vi "excelBinDataMT1.vi"(5 "step":string, 6 "start row":i32, 7 "jobno":string, 8 "error in (no error) 2":errorcluster, 9 "report in":refnum<class "NI_report.lvclass">, 10 "error in (no error)":errorcluster, 11 "connection reference 2":T1) -> (0 "error out 2":errorcluster, 1 "report out":refnum<class "NI_report.lvclass">, 2 "error out":errorcluster, 3 "connection reference":T1)   [LabVIEW 2012]
uses:
  <vilib>/addons/database/Connection.llb/Conn ObjectReference.ctl
  <vilib>/Utility/NIReport.llb/NI_report.lvclass
  <vilib>/addons/database/Auxilliary.llb/DB Tools Cursor Type.ctl
  <vilib>/addons/database/Connection.llb/Conn Execute.vi
  <vilib>/addons/database/Recordset.llb/Rec Fetch String Data (R).vi
  <vilib>/addons/database/Recordset.llb/Rec Fetch Integer Data (R).vi
  <vilib>/addons/database/Recordset.llb/Rec Destroy - Connection.vi
  <vilib>/addons/database/NI_Database_API.lvlib
  <vilib>/Utility/NIReport.llb/Excel/NI_Excel.lvclass
panel:
  in  "start (0, 0)":cluster{"start row":i32, "start column":i32}
  out "concatenated string":string
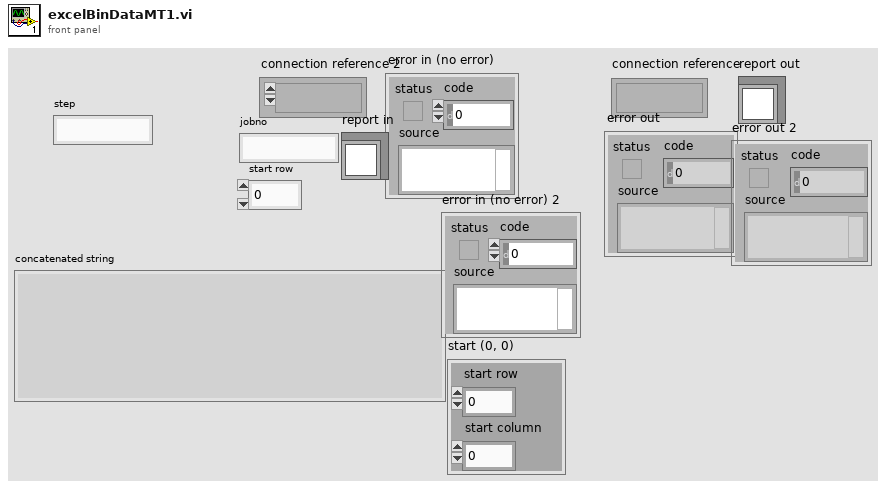
[diagram p1: front panel]
types:
  T1 = typedef "NI_Database_API.lvlib/Conn ObjectReference.ctl" = refnum<k1>
  T2 = typedef "NI_Database_API.lvlib/DB Tools Cursor Type.ctl" = enum16{"forward-only", "keyset", "dynamic", "static"}
  T3 = typedef "NI_Database_API.lvlib/Rec ObjectReference.ctl" = refnum<k1>
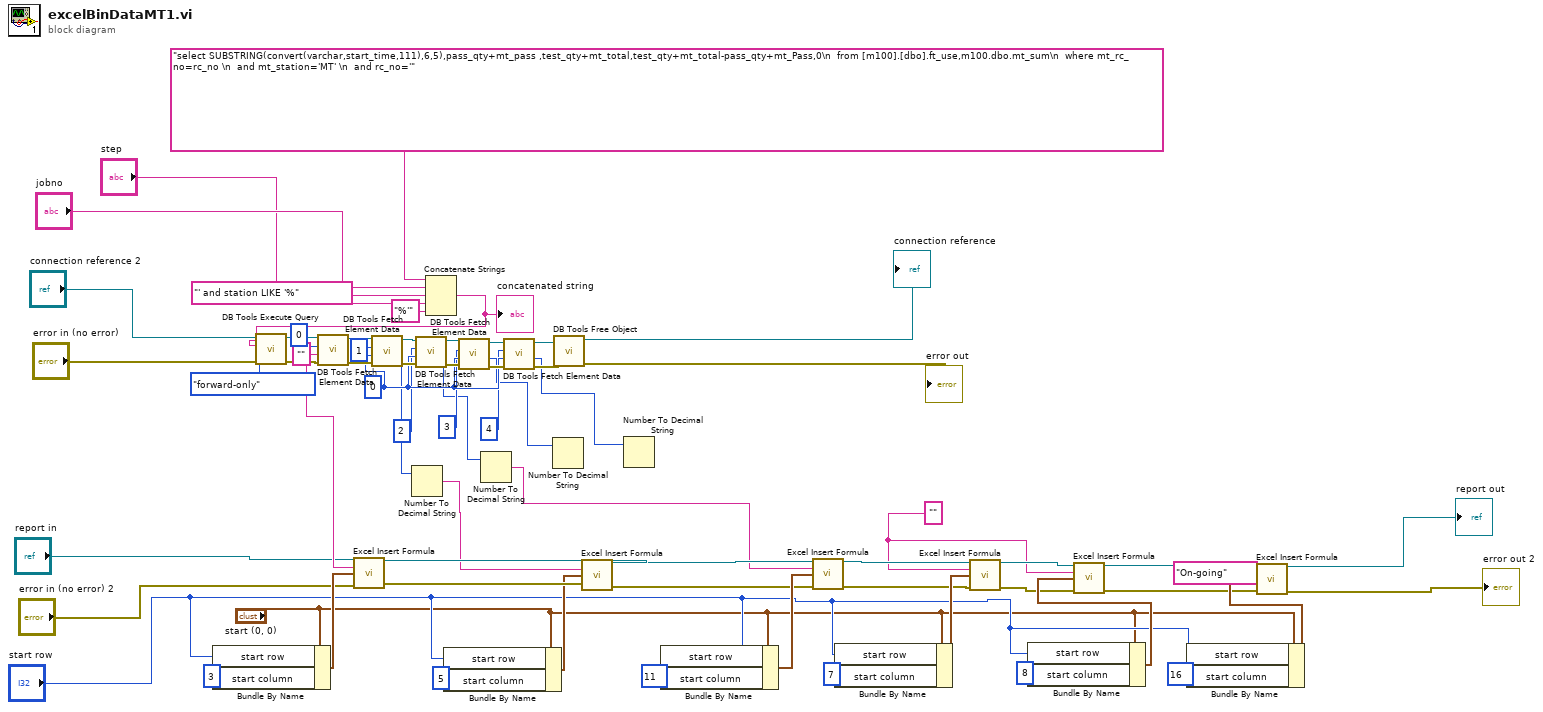
[diagram p0: block diagram]
diagram:
  w1 = "" ("formula")
  w49 = 0
  n1 = Bundle By Name(cluster="start (0, 0)", "start row"="start row", "start column"=3) -> (w44:cluster{"start row":i32, "start column":i32})
  n2 = Concatenate Strings("select SUBSTRING(convert(varchar,start_time,111),6,5),pass_qty+mt_pass ,test_qty+mt_total,test_qty+mt_total-pass_qty+mt_Pass,0\n  from [m100].[dbo].ft_use,m100.dbo.mt_sum\n  where mt_rc_no=rc_no \n  and mt_station='MT' \n  and rc_no='", "jobno", "' and station LIKE '%" ("string"), "step", "%'" ("string")) -> (w65:string)
  "concatenated string" <- w65
  n3 = call-poly <vilib>:"DB Tools Execute Query.vi"("error in (no error)"="error in (no error)", "cursor type"=DB_Tools_Cursor_Type."forward-only", "SQL query"=w65, "connection reference"="connection reference 2") -> ("error out"=w62:errorcluster, "recordset reference"=w63:T3)  [unwired: 4 in]
  n4 = call-poly <vilib>:"DB Tools Fetch Element Data.vi"("error in (no error)"=w62, "type"="", "column index"=0, "recordset reference"=w63) -> ("error out"=w58:errorcluster, "data"=w43:string, "recordset reference out"=w59:T3)  [unwired: 3 in]
  n5 = call <vilib>:"Excel Insert Formula.vi"("report in"="report in", "formula"=w43, "start (0, 0)"=w44, "error in (no error)"="error in (no error) 2") -> ("report out"=w41:refnum<class "NI_report.lvclass">, "error out"=w40:errorcluster)  [unwired: 10 in]
  n6 = call-poly <vilib>:"DB Tools Fetch Element Data.vi"("error in (no error)"=w58, "type"=w49, "column index"=1, "recordset reference"=w59) -> ("error out"=w53:errorcluster, "data"=w38:i32, "recordset reference out"=w57:T3)  [unwired: 3 in]
  n7 = Number To Decimal String(number=w38) -> (decimal integer string=w37:string)  [unwired: 1 in]
  n8 = call-poly <vilib>:"DB Tools Fetch Element Data.vi"("error in (no error)"=w53, "type"=w49, "column index"=2, "recordset reference"=w57) -> ("error out"=w52:errorcluster, "data"=w31:i32, "recordset reference out"=w56:T3)  [unwired: 3 in]
  n9 = Bundle By Name(cluster="start (0, 0)", "start row"="start row", "start column"=5) -> (w36:cluster{"start row":i32, "start column":i32})
  n10 = call-poly <vilib>:"DB Tools Fetch Element Data.vi"("error in (no error)"=w52, "type"=w49, "column index"=3, "recordset reference"=w56) -> ("error out"=w51:errorcluster, "data"=w29:i32, "recordset reference out"=w55:T3)  [unwired: 3 in]
  n11 = Number To Decimal String(number=w31) -> (decimal integer string=w30:string)  [unwired: 1 in]
  n12 = call-poly <vilib>:"DB Tools Fetch Element Data.vi"("error in (no error)"=w51, "type"=w49, "column index"=4, "recordset reference"=w55) -> ("error out"=w50:errorcluster, "data"=w28:i32, "recordset reference out"=w54:T3)  [unwired: 3 in]
  n13 = Number To Decimal String(number=w29) -> ()  [unwired: 1 in, 1 out]
  n14 = call-poly <vilib>:"DB Tools Free Object.vi"("error in (no error)"=w50, "recordset reference"=w54) -> ("error out"=→"error out":errorcluster, "connection reference"=→"connection reference":T1)  [unwired: 8 in]
  n15 = call <vilib>:"Excel Insert Formula.vi"("report in"=w41, "formula"=w37, "start (0, 0)"=w36, "error in (no error)"=w40) -> ("report out"=w32:refnum<class "NI_report.lvclass">, "error out"=w34:errorcluster)  [unwired: 10 in]
  n16 = Number To Decimal String(number=w28) -> ()  [unwired: 1 in, 1 out]
  n17 = Bundle By Name(cluster="start (0, 0)", "start row"="start row", "start column"=11) -> (w35:cluster{"start row":i32, "start column":i32})
  n18 = call <vilib>:"Excel Insert Formula.vi"("report in"=w32, "formula"=w30, "start (0, 0)"=w35, "error in (no error)"=w34) -> ("report out"=w23:refnum<class "NI_report.lvclass">, "error out"=w21:errorcluster)  [unwired: 10 in]
  n19 = Bundle By Name(cluster="start (0, 0)", "start row"="start row", "start column"=7) -> (w25:cluster{"start row":i32, "start column":i32})
  n20 = call <vilib>:"Excel Insert Formula.vi"("report in"=w23, "formula"=w1, "start (0, 0)"=w25, "error in (no error)"=w21) -> ("report out"=w22:refnum<class "NI_report.lvclass">, "error out"=w20:errorcluster)  [unwired: 10 in]
  n21 = Bundle By Name(cluster="start (0, 0)", "start row"="start row", "start column"=8) -> (w24:cluster{"start row":i32, "start column":i32})
  n22 = call <vilib>:"Excel Insert Formula.vi"("report in"=w22, "formula"=w1, "start (0, 0)"=w24, "error in (no error)"=w20) -> ("report out"=w5:refnum<class "NI_report.lvclass">, "error out"=w6:errorcluster)  [unwired: 10 in]
  n23 = Bundle By Name(cluster="start (0, 0)", "start row"="start row", "start column"=16) -> (w7:cluster{"start row":i32, "start column":i32})
  n24 = call <vilib>:"Excel Insert Formula.vi"("report in"=w5, "formula"="On-going", "start (0, 0)"=w7, "error in (no error)"=w6) -> ("report out"=→"report out":refnum<class "NI_report.lvclass">, "error out"=→"error out 2":errorcluster)  [unwired: 10 in]
